vi "LineParser.vi"(1 "Line String":string) -> (0 "output array":string[](array[string]))   [LabVIEW 2014]
panel:
  out "index":i32
  out "quote":bool
  out "token":string
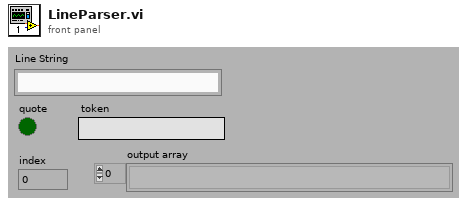
[diagram p1: front panel]
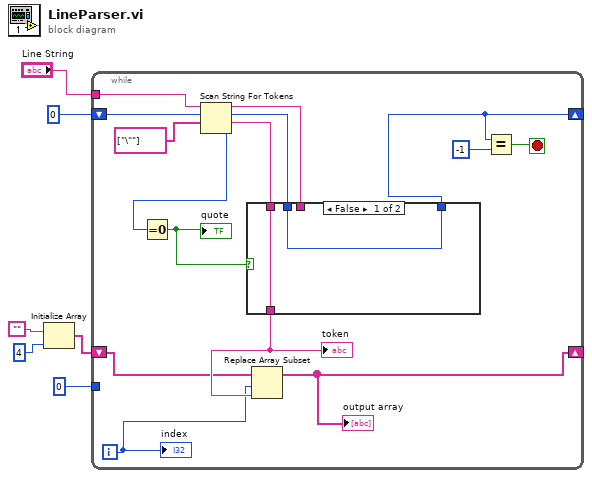
[diagram p0: block diagram]
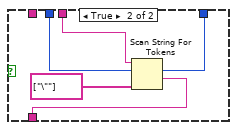
[diagram p2: hidden frame]
diagram:
  n1 = Initialize Array("", 4 ("dimension size")) -> (w1:string[])
  n2 = while {
    tunnel: "Line String" -> [w21]
    shift-right: [w12] -> _
    shift-left: 0 ("offset past token") -> [w20]
    tunnel: 0 -> [_]
    shift-right: [w8] -> _
    shift-left: w1 -> [w9]
    i -> [w7]
    stop <- w19 stop-if-true
    n3 = Scan String For Tokens(7:string[] ["\""] ("operators (none)"), 8:w20, 9:w21) -> (0:w18:i32, 1:w13:string, 2:w14:i32, 3:w16:string)  [unwired: 3 in]
    n4 = Equal To 0?(x=w18) -> (x = 0?=w15:bool)
    "quote" <- w15
    n5 = case shown="False" w15 {
      tunnel: w14 -> [w23 w25]
      tunnel: w16 -> [_ w27]
      tunnel: [w23 w26] -> w12
      tunnel: w13 -> [w22 _]
      tunnel: [w22 w24] -> w10
      frame False {
      }
      frame True {
        n6 = Scan String For Tokens(6:string[] ["\""] ("delimiters (\\s,\\t,\\r,\\n)"), 8:w25, 9:w27) -> (1:w24:string, 2:w26:i32)  [unwired: 3 in, 2 out]
      }
    }
    "token" <- w10
    n7 = Replace Array Subset(array=w9, new element=w10, index=w7) -> (w8:string[])
    "output array" <- w8
    n8 = Equal?(x=w12, y=-1) -> (x = y?=w19:bool)
    "index" <- w7
  }
